vi "TDC_releaseLftFunction.vi"(8 "Error In":errorcluster, 11 "Function":u64) -> (0 "Error Out":errorcluster)   [LabVIEW 2011]
uses:
  tdcbase.dll
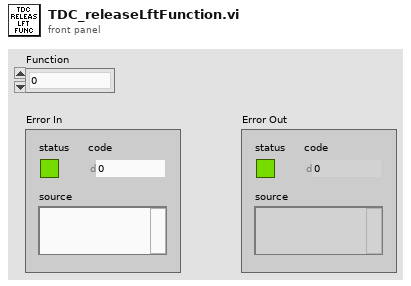
[diagram p1: front panel]
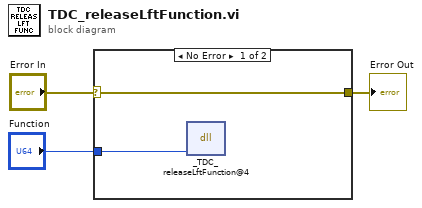
[diagram p0: block diagram]
diagram:
  n1 = case shown="No Error" "Error In" {
    selector: "Error In" -> [w5 w6]
    tunnel: [w5 w6] -> w2
    tunnel: "Function" -> [w4 _]
    frame No Error {
      n2 = dll-call lib="X:/tdcbase.dll" fn="_TDC_releaseLftFunction@4"("function"=w4) -> ()  [unwired: 5 in, 2 out]
    }
    frame Error {
    }
  }
  "Error Out" <- w2
